vi "10-Tap 8-bit Camera without DRAM (FPGA-SIM)RandomSimDataNoHostDMAs.vi"() -> ()   [LabVIEW 2013]
doc: "This is the FPGA VI for the 10-Tap 8-Bit Camera with DRAM example. This example demonstrates how to acquire images from a 10-tap, 8-bit, extended configuration, Camera Link camera and transfer the images to the host. This example supports area scan and line scan cameras for both continuous and finite acquisitions.\n\nThis example also demonstrates the use of DRAM as a frame buffer for very high speed acquisitions. Data packing and flow-control are also employed to maximize use of the available DRAM and FIFOs in terms of both memory space and performance.\n\nAdditionally, the example demonstrates the serial server, which allows third-party camera configuration utilities to communicate with the camera using the Camera Link serial interface while this VI is running."
uses:
  Common/CL Signal Mapping.ctl
  Common/CL Configuration.ctl
  FPGA/Sector/Accumulate/Sector Parameter Cluster.ctl
  <vilib>/Platform/TimedLoop/XDataNode/timing_clust.ctl
  <vilib>/Platform/TimedLoop/XDataNode/nitl_modes.ctl
  <vilib>/Platform/TimedLoop/XDataNode/wakeup.ctl
  <vilib>/rvi/Emulation/niFpgaSctlEmulationGetInTimedLoop.vi
  <vilib>/rvi/Emulation/niFpgaEmulationReportErrorSimple.vi
  <vilib>/rvi/Emulation/niFpgaGetClockAttributes.vi
  <vilib>/rvi/Emulation/niFpgaCriticalErrorInLSC.vi
  <vilib>/rvi/FIFO/Fifo_Resource/nirvififoEmulationGetNumberOfElementsToWriteFpgaImpl.vi
  <vilib>/rvi/DataTransferAndStorage/Container/Common/niFpgaContainerGetUniqueNameForEmu.vi
  <vilib>/rvi/FIFO/Fifo_Resource/nirvififoEmulationWriteFpgaImpl.vi
  <vilib>/rvi/FIFO/Fifo_Resource/nirvififoEmulationGetNumberOfElementsToReadFpgaImpl.vi
  <vilib>/rvi/FIFO/Fifo_Resource/nirvififoEmulationReadFpgaImpl.vi
  <vilib>/rvi/Emulation/niFpgaProcessEmulError.vi
  FPGA/Globals/Pixel Location Global.vi
  FPGA/Globals/Sector Parameter Global.vi
  FPGA/Globals/Accumulated Sector Intensity.vi
  <vilib>/Platform/TimedLoop/XDataNode/XDataNode.xnode
  <vilib>/rvi/DataTransferAndStorage/Container/XNode/niFpgaContainer.xnode
  <vilib>/rvi/FIFO/Fifo_Resource/nirvififoEmulationGetNumberOfElementsToWrite.vi
  <vilib>/rvi/FIFO/Fifo_Resource/nirvififoEmulationWrite.vi
  <vilib>/rvi/FIFO/Fifo_Resource/nirvififoEmulationGetNumberOfElementsToRead.vi
  <vilib>/rvi/FIFO/Fifo_Resource/nirvififoEmulationRead.vi
  <vilib>/Platform/TimedLoop/XDataNode/XDNodeRunTimeDep.lvlib
  FPGA/Globals/Wing Square Wave Frequency Global.vi
panel:
  in  "Sim Data":u64=44
  out "Number of Elements to Write Sector Grouping FIFO":u32
  out "Accumulate Ticks":u32
  out "Analysis Ticks":u32
  out "Target Sim TO":bool
  out "Cam Data Timeout":bool
  out "Sector FIFO Timeout":bool
  out "Host DMA Timeout":bool
  out "Number of Elements to Read Cam Data":u32
  out "Number of Elements to Write Host DMA":u32
  in  "Words per image":u32=1000
  in  "Y Resolution":u16=1000
  in  "X Resolution":u16=1000
  in  "[Average BG Intensity]":u8[](array[numeric])=[0, 0, 0, 0, 0, 0, 0, 0, 0, 0, 0, 0, 0, 0, 0, 0, 0, 0, 0, 0, 0, 0, 0, 0, 0, 0, 0, 0, 0, 0, 0, 0]
  in  "Sector Threshold":u8
  in  "# of Frames to Average":u8=1
  in  "Sector Parameters Right":T1={"Start Angle"=0.0, "End Angle"=0.4708251953125, "Inner Radius"=309, "Outter Radius"=405, "Hinge X"=685, "Hinge Y"=527, "NumWingSectors"=8}
  in  "Sector Parameters Left":T1={"Start Angle"=0.65740966796875, "End Angle"=0.99468994140625, "Inner Radius"=309, "Outter Radius"=405, "Hinge X"=464, "Hinge Y"=534, "NumWingSectors"=8}
  in  "CL Config.Configuration":T2=enum."Full"
  in  "CL Config.Signal Mapping":T3=enum."Basler 10-tap"
  in  "CL Config.Line Scan":bool
  in  "CL Config.DVAL Active High":bool=TRUE
  in  "CL Config.LVAL Active High":bool=TRUE
  in  "CL Config.FVAL Active High":bool=TRUE
  in  "CL Config.Spare Active High":bool=TRUE
  in  "Acq Control.Line Scan Height":u32
  in  "Acq Control.Frames To Acq":u32
  in  "Acq Control.Acquire":bool
  in  "Acq Control.Cancel Acq":bool
  in  "Acq Control.Ignore DVAL":bool
  in  "Acq Control.Initialize":bool
  out "Acq Status.Acq In Progress":bool
  out "Acq Status.Clocks Per Line":u32
  out "Acq Status.Frames Acq'd":u32
  out "Acq Status.Lines Per Frame":u32
  out "Acq Status.DMA Write Timeout":bool
  out "Acq Status.Initialized":bool
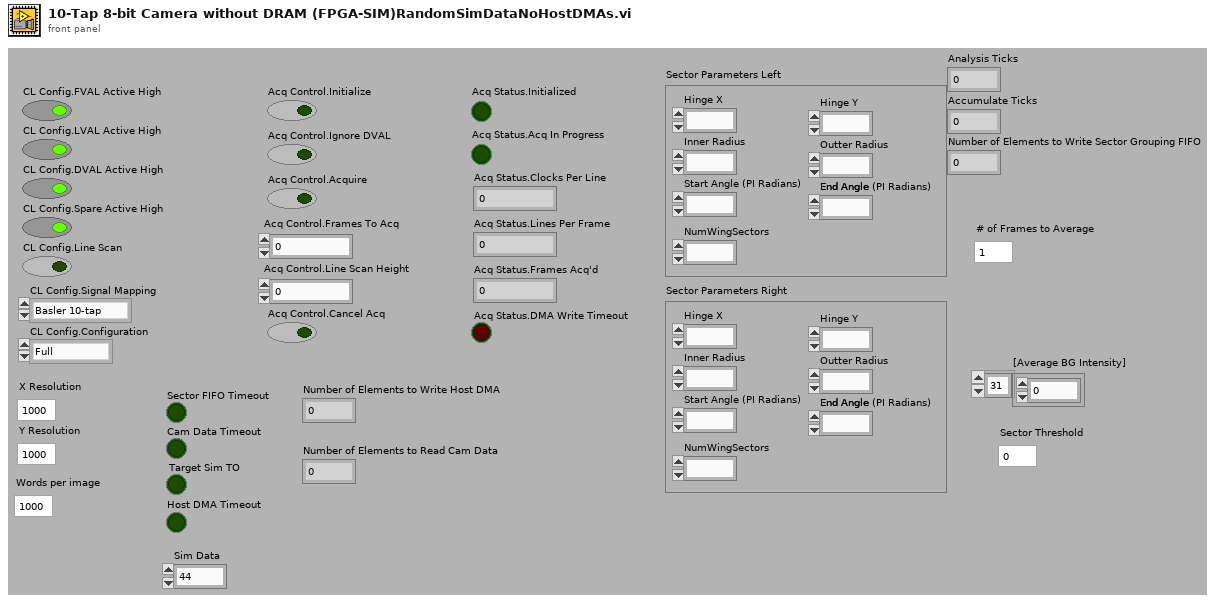
[diagram p1: front panel]
types:
  T1 = typedef "Sector Parameter Cluster.ctl" = cluster{"Start Angle":fxp<+/-,17,2>, "End Angle":fxp<+,17,3>, "Inner Radius":u16, "Outter Radius":u16, "Hinge X":u16, "Hinge Y":u16, "NumWingSectors":u8}
  T2 = typedef "CL Configuration.ctl" = enum8{"Base", "Medium", "Full"}
  T3 = typedef "CL Signal Mapping.ctl" = enum8{"Standard", "Basler 10-tap", "Vosskühler 10-tap"}
  T4 = typedef "XDNodeRunTimeDep.lvlib/timing_clust.ctl" = cluster{"Expected End [f-1]":u64, "Actual End [f-1]":u64, "Finished Late? [f-1]":bool, "Expected End [i-1]":u64, "Actual End [i-1]":u64, "Finished Late? [i-1]":bool, "Expected Start [i]":u64, "Actual Start [i]":u64, "Expected Start [f]":u64, "Actual Start [f]":u64, "Source Name":string, "Structure Name":string, "Period":i64, "Deadline":i64, "Offset":i64, "Start":i64, "Priority":i32, "Timeout":i32, "Mode":T5, "Wakeup Reason":T6, "Error":errorcluster, "Source Type":string, "Secondary Source Type":string, "Global End Time":u64, "Global Start Time":u64, "Frame Duration":u64, "Iteration Duration":u64, "Assigned CPU":i32, "I/O Scan Engine Mode":u32}
  T5 = typedef "XDNodeRunTimeDep.lvlib/nitl_modes.ctl" = enum32{"No Change", "Process missed periods, maintain original phase", "Discard missed periods, maintain original phase", "Process missed periods, ignore original phase", "Discard missed periods, ignore original phase"}
  T6 = typedef "XDNodeRunTimeDep.lvlib/wakeup.ctl" = enum32{"Normal", "Aborted", "Asynchronous wakeup", "Timing source error", "Timed loop error", "Timeout"}
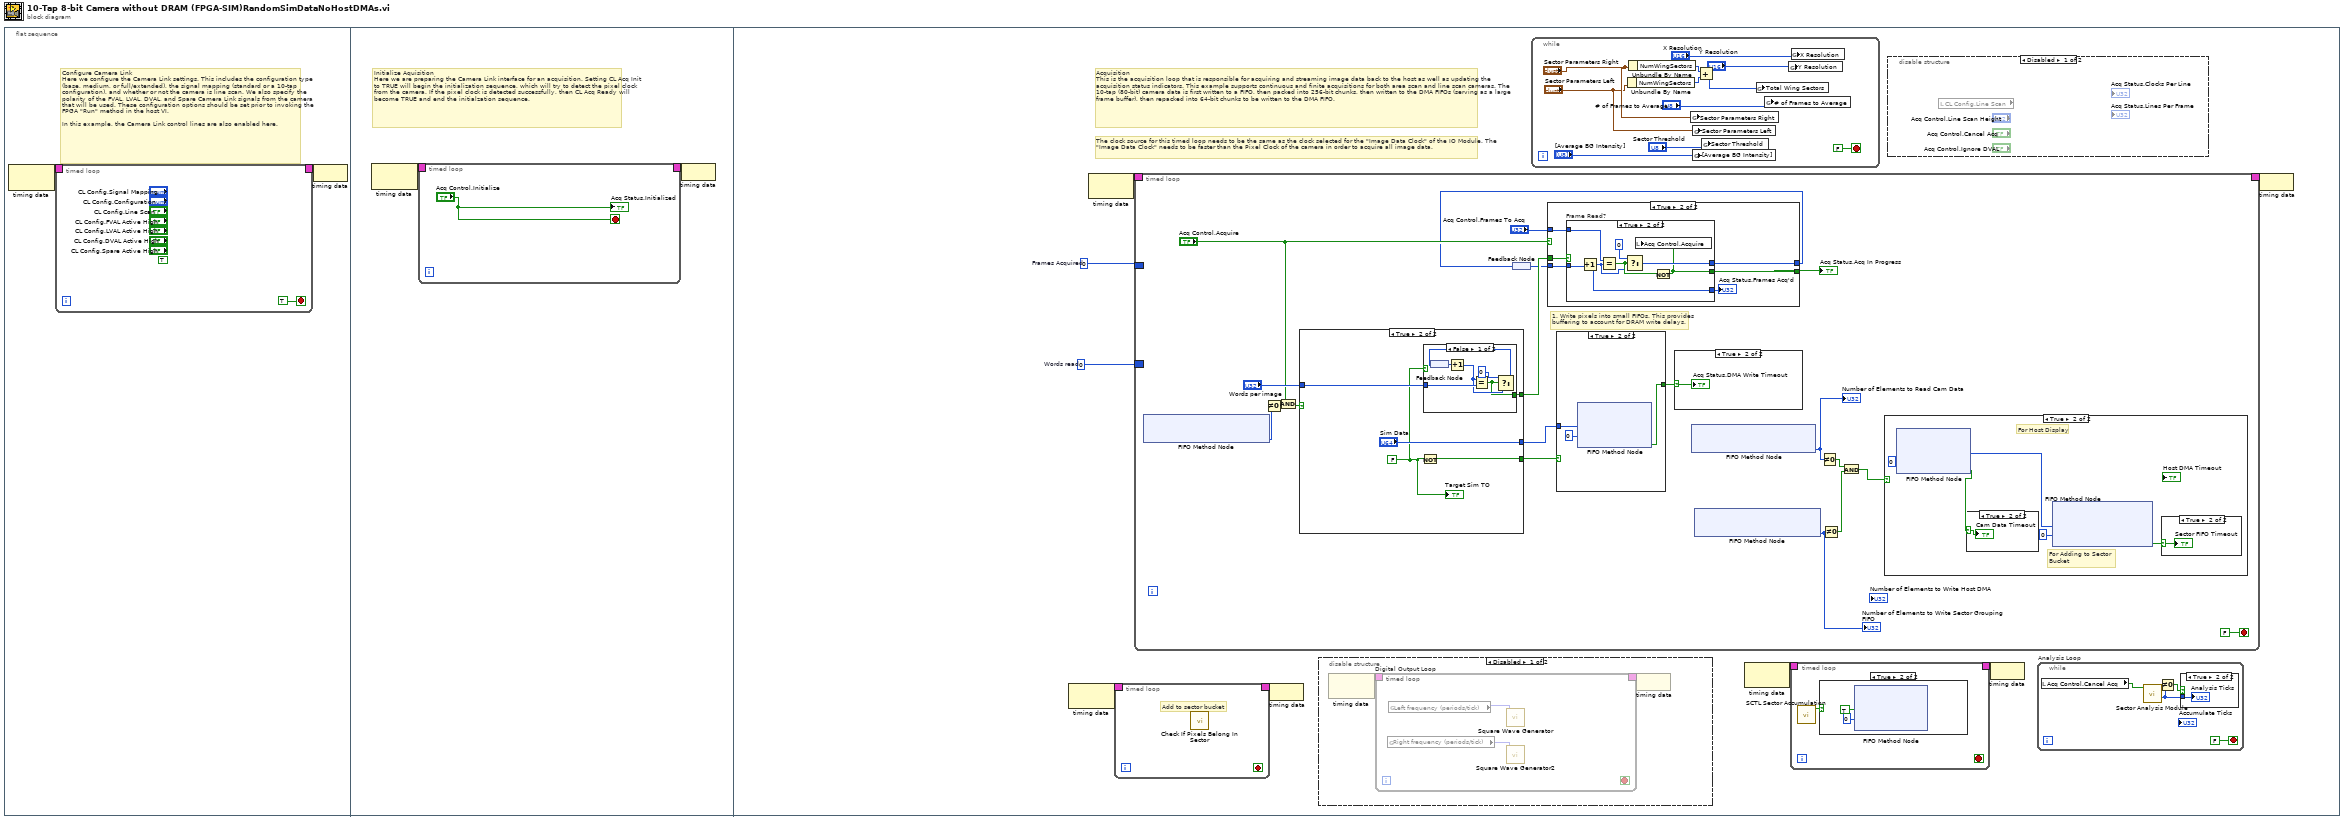
[diagram p0: block diagram]
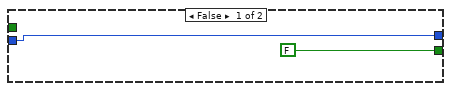
[diagram p7: hidden frame]
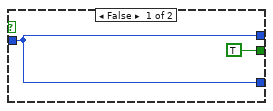
[diagram p8: hidden frame]
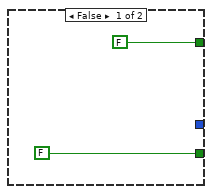
[diagram p9: hidden frame]
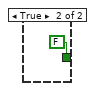
[diagram p10: hidden frame]
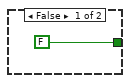
[diagram p14: hidden frame]
diagram:
  n1 = flat-sequence {
    frame #0 {
      # "Configure Camera Link\nHere we configure the Camera Link settings. This includes the configuration type (base, medium, or full/extended), the signal mapping (standard or a 10-tap configuration), and whether or not the camera is line scan. We also specify the polarity of the FVAL, LVAL, DVAL, and Spare Camera Link signals from the camera that will be used. These configuration options should be set prior to invoking the FPGA \"Run\" method in the host VI.\n\nIn this example, the Camera Link control lines are also enabled here."
      n2 = node-c288() -> (w2:T4)  [unwired: 1 in]
      n3 = timed-loop {
        timing: w2 -> [_]
        timing-out: [_] -> w1
        stop <- TRUE stop-if-true
        (unwired) TRUE ("IO Module\\CL Control Enable")
      }
      n4 = node-c288(w1) -> ()
    }
    frame #1 {
      # "Initialize Aquisition\nHere we are preparing the Camera Link interface for an acquisition. Setting CL Acq Init to TRUE will begin the initialization sequence, which will try to detect the pixel clock from the camera. If the pixel clock is detected successfully, then CL Acq Ready will become TRUE and end the initialzation sequence."
      n5 = node-c288() -> (w9:T4)  [unwired: 1 out]
      n6 = timed-loop {
        timing: w9 -> [_]
        timing-out: [_] -> w8
        stop <- "Acq Control.Initialize" stop-if-true
        "Acq Status.Initialized" <- "Acq Control.Initialize"
      }
      n7 = node-c288(w8) -> ()
    }
    frame #2 {
      w19 = u32 0  # Frames Acquired
      w20 = u32 0  # Words read
      # "The clock source for this timed loop needs to be the same as the clock selected for the \"Image Data Clock\" of the IO Module. The \"Image Data Clock\" needs to be faster than the Pixel Clock of the camera in order to acquire all image data."
      # "Acquisition\nThis is the acquisition loop that is responsible for acquiring and streaming image data back to the host as well as updating the acquisition status indicators. This example supports continuous and finite acquisitions for both area scan and line scan cameras. The 10-tap (80-bit) camera data is first written to a FIFO, then packed into 256-bit chunks, then written to the DMA FIFOs (serving as a large frame buffer), then repacked into 64-bit chunks to be written to the DMA FIFO."
      n8 = node-c288() -> (w16:T4)  [unwired: 1 in]
      n9 = node-c288() -> (w22:T4)  [unwired: 1 in]
      n10 = timed-loop {
        timing: w16 -> [_]
        timing-out: [_] -> w15
        stop <- _ stop-if-true
        # "Add to sector bucket"
        n11 = call "Check If Pixels Belong In Sector.vi"() -> ()  [unwired: 11 in, 1 out]
      }
      n12 = timed-loop {
        timing: w22 -> [_]
        timing-out: [_] -> w21
        border: w20 -> [_]
        border: w19 -> [_]
        stop <- FALSE stop-if-true
        # "1. Write pixels into small FIFOs. This provides\nbuffering to account for DRAM write delays."
        n13 = xnode ("FIFO Method Node")() -> ("Number of Elements to Write"=w61:u32)  [unwired: 1 in, 1 out]
        n14 = Not Equal To 0?(x=w61) -> (x != 0?=w60:bool)
        n15 = Compound Arithmetic op=AND("Acq Control.Acquire", w60) -> (w66:bool)
        n16 = case shown="True" w66 {
          tunnel: [_ "Sim Data"] -> w70
          tunnel: [FALSE w93] -> w68
          tunnel: "Words per image" -> [_ w95]
          tunnel: [FALSE w94] -> w57
          frame False {
          }
          frame True {
            w91 = FALSE ("x")
            n17 = Not(x=w91) -> (.not. x?=w93:bool)
            n18 = case shown="False" w91 {
              tunnel: w95 -> [w101 _]
              tunnel: [w96 FALSE] -> w94
              frame False {
                n19 = feedback #1() -> (w100:u32)
                n20 = Increment(x=w100) -> (x+1=w97:u32)
                n21 = Equal?(x=w97, y=w101) -> (x = y?=w96:bool)
                n22 = Select(t=u32 0 ("Acq Status.Frames Acq'd"), s=w96, f=w97) -> (s? t:f=w98:u32)
                n23 = feedback-in #1(w98) -> ()
              }
              frame True {
              }
            }
            "Target Sim TO" <- w91
          }
        }
        n24 = feedback #2() -> (w56:u32)
        n25 = case shown="True" "Acq Control.Acquire" {
          tunnel: w57 -> [_ w79]
          tunnel: w56 -> [w73 w78]
          tunnel: "Acq Control.Frames To Acq" -> [_ w77]
          tunnel: [w73 w76] -> w54
          tunnel: [FALSE w75] -> w53
          frame False {
          }
          frame True {
            n26 = case "Frame Read?" shown="True" w79 {
              tunnel: w78 -> [w80 w88]
              tunnel: w77 -> [_ w87]
              tunnel: [w80 w85] -> w76
              tunnel: [TRUE w83] -> w75
              tunnel: [w80 w82] -> w74
              frame False {
              }
              frame True {
                n27 = Increment(x=w88) -> (x+1=w82:u32)
                n28 = Equal?(x=w87, y=w82) -> (x = y?=w84:bool)
                n29 = Select(t=u32 0 ("Frames Acquired"), s=w84, f=w82) -> (s? t:f=w85:u32)
                n30 = Not(x=w84) -> (.not. x?=w83:bool)
                n31 = local write "Acq Control.Acquire"(w83) -> ()
              }
            }
            "Acq Status.Frames Acq'd" <- w74
          }
        }
        "Acq Status.Acq In Progress" <- w53
        n32 = feedback-in #2(w54) -> ()
        n33 = case shown="True" w68 {
          tunnel: [FALSE ("Timed Out?") w112] -> w52
          tunnel: w70 -> [_ w113]
          frame False {
          }
          frame True {
            n34 = xnode ("FIFO Method Node")("Element"=w113, "Timeout"=0) -> ("Timed Out?"=w112:bool)  [unwired: 1 in, 1 out]
          }
        }
        n35 = case shown="True" w52 {
          selector: w52 -> [_ w71]
          frame False {
          }
          frame True {
            "Acq Status.DMA Write Timeout" <- w71
          }
        }
        n36 = xnode ("FIFO Method Node")() -> ("Number of Elements to Read"=w63:u32)  [unwired: 1 in, 1 out]
        "Number of Elements to Read Cam Data" <- w63
        n37 = xnode ("FIFO Method Node")() -> ("Number of Elements to Write"=w65:u32)  [unwired: 1 in, 1 out]
        "Number of Elements to Write Sector Grouping FIFO" <- w65
        n38 = Not Equal To 0?(x=w63) -> (x != 0?=w62:bool)
        n39 = Not Equal To 0?(x=w65) -> (x != 0?=w64:bool)
        n40 = Compound Arithmetic op=AND(w62, w64) -> (w67:bool)
        n41 = case shown="True" w67 {
          frame False {
          }
          frame True {
            # "For Adding to Sector \nBucket"
            # "For Host Display"
            n42 = xnode ("FIFO Method Node")("Timeout"=0) -> ("Element"=w106:u64, "Timed Out?"=w103:bool)  [unwired: 1 in, 1 out]
            n43 = case shown="True" w103 {
              selector: w103 -> [_ w108]
              frame False {
              }
              frame True {
                "Cam Data Timeout" <- w108
              }
            }
            n44 = xnode ("FIFO Method Node")("Element"=w106, "Timeout"=0) -> ("Timed Out?"=w104:bool)  [unwired: 1 in, 1 out]
            n45 = case shown="True" w104 {
              selector: w104 -> [_ w109]
              frame False {
              }
              frame True {
                "Sector FIFO Timeout" <- w109
              }
            }
          }
        }
      }
      n46 = node-c288(w15) -> ()
      n47 = disable-structure shown="Disabled" {
        frame Disabled {
          n48 = node-c288() -> (w35:T4)  [unwired: 1 in]
          n49 = timed-loop "Digital Output Loop" {
            timing: w35 -> [_]
            timing-out: [_] -> w34
            stop <- _ stop-if-true
            n50 = global read "Wing Square Wave Frequency Global.vi" "Right frequency (periods/tick)"() -> (w36:fxp<+,32,0>)
            n51 = global read "Wing Square Wave Frequency Global.vi" "Left frequency (periods/tick)"() -> (w37:fxp<+,32,0>)
            n52 = call "Square Wave Generator"("frequency (periods/tick)"=w37) -> ()  [unwired: 14 in, 1 out]
            n53 = call "Square Wave Generator2"("frequency (periods/tick)"=w36) -> ()  [unwired: 14 in, 1 out]
          }
          n54 = node-c288(w34) -> ()
        }
        frame Enabled {
        }
      }
      n55 = while {
        stop <- FALSE stop-if-true
        n56 = Unbundle By Name("Sector Parameters Left") -> ("NumWingSectors"=w126:u8)
        n57 = Unbundle By Name("Sector Parameters Right") -> ("NumWingSectors"=w127:u8)
        n58 = global write "Sector Parameter Global.vi" "Sector Parameters Right"("Sector Parameters Right") -> ()
        n59 = global write "Sector Parameter Global.vi" "Sector Parameters Left"("Sector Parameters Left") -> ()
        n60 = global write "Sector Parameter Global.vi" "[Average BG Intensity]"("[Average BG Intensity]") -> ()
        n61 = Add(x=w127, y=w126) -> (x+y=w125:u8)
        n62 = global write "Sector Parameter Global.vi" "Sector Threshold"("Sector Threshold") -> ()
        n63 = global write "Accumulated Sector Intensity.vi" "Total Wing Sectors"(w125) -> ()
        n64 = global write "Pixel Location Global.vi" "# of Frames to Average"("# of Frames to Average") -> ()
        n65 = global write "Pixel Location Global.vi" "Y Resolution"("Y Resolution") -> ()
        n66 = global write "Pixel Location Global.vi" "X Resolution"("X Resolution") -> ()
      }
      n67 = node-c288() -> (w18:T4)  [unwired: 1 in]
      n68 = timed-loop {
        timing: w18 -> [_]
        timing-out: [_] -> w17
        stop <- _ stop-if-true
        n69 = call "SCTL Sector Accumulation.vi"() -> ("New Data?"=w27:bool)  [unwired: 11 in]
        n70 = case shown="True" w27 {
          frame False {
          }
          frame True {
            n71 = xnode ("FIFO Method Node")("Element"=TRUE, "Timeout"=0) -> ()  [unwired: 1 in, 2 out]
          }
        }
      }
      n72 = disable-structure shown="Disabled" {
        frame Disabled {
          n73 = local read "CL Config.Line Scan"() -> (w44:bool)
        }
        frame Enabled {
        }
      }
      n74 = node-c288(w17) -> ()
      n75 = while "Analysis Loop" {
        stop <- FALSE stop-if-true
        n76 = local read "Acq Control.Cancel Acq"() -> (w49:bool)
        n77 = call "Sector Analysis Module.vi"("Canceled?"=w49) -> ("Analysis Ticks"=w48:u32)  [unwired: 8 in, 2 out]
        n78 = Not Equal To 0?(x=w48) -> (x != 0?=w47:bool)
        n79 = case shown="True" w47 {
          tunnel: w48 -> [_ w51]
          frame False {
          }
          frame True {
            "Analysis Ticks" <- w51
          }
        }
      }
      n80 = node-c288(w21) -> ()
    }
  }
